vi "Thermometer Reading with Warning LED.vi"() -> ()   [LabVIEW 2020]
panel:
  out "Waveform Chart":T1(graph)
  in  "stop":bool
  out "WARNING":bool
  in  "LOW Limit":dbl
  in  "HIGH Limit":dbl
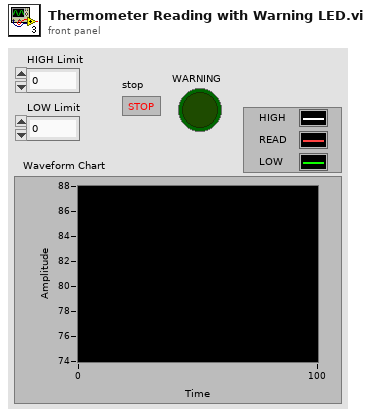
[diagram p1: front panel]
types:
  T1 = cluster{"HIGH Limit":dbl, "Reading (degC)":dbl, "LOW Limit":dbl}
  T2 = cluster{"HIGH Limit":dbl, "Temperature (deg F)":dbl, "LOW Limit":dbl}
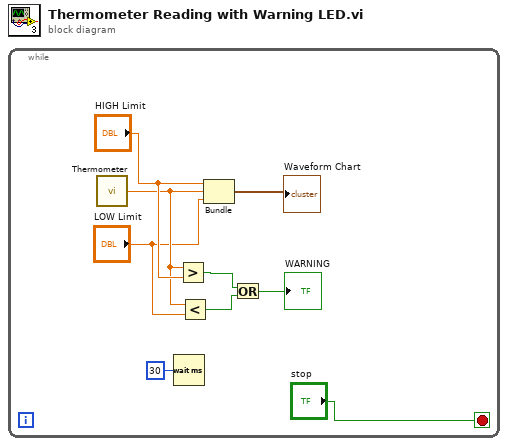
[diagram p0: block diagram]
diagram:
  n1 = while {
    stop <- "stop" stop-if-true
    n2 = call "Thermometer.vi"() -> ("Temperature (deg F)"=w7:dbl)  [unwired: 1 in]
    n3 = Wait (ms)(milliseconds to wait=u32 30) -> ()  [unwired: 1 out]
    n4 = Greater?(x=w7, y="HIGH Limit") -> (0:w3:bool)
    n5 = Less?(x=w7, y="LOW Limit") -> (x < y?=w5:bool)
    n6 = Bundle("HIGH Limit"="HIGH Limit", "Temperature (deg F)"=w7, "LOW Limit"="LOW Limit") -> (→"Waveform Chart":T2)  [unwired: 1 in]
    n7 = Or(x=w3, y=w5) -> (x .or. y?=→"WARNING":bool)
  }
